vi "Read GMaps Attributes.vi"(0 "GMaps API in":refnum<class "GMaps API.lvclass">, 5 "error in (no error)":errorcluster) -> (14 "GMaps API out":refnum<class "GMaps API.lvclass">, 15 "GMaps Attributes":T1, 19 "error out":errorcluster)   [LabVIEW 2016, in "GMaps API.lvclass"]
doc: "Reads GMaps configured request."
uses:
  GMaps API.lvclass
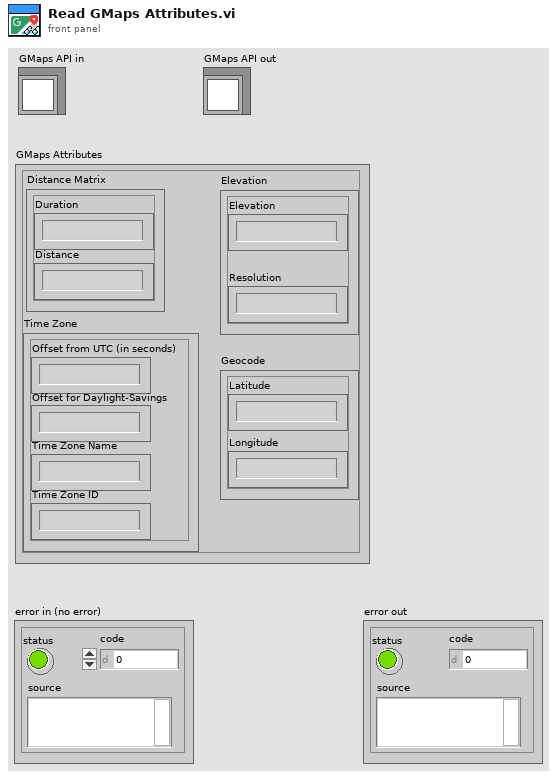
[diagram p1: front panel]
types:
  T1 = cluster{"Distance Matrix":cluster{"Duration":string, "Distance":string}, "Time Zone":cluster{"Offset from UTC (in seconds)":string, "Offset for Daylight-Savings":string, "Time Zone Name":string, "Time Zone ID":string}, "Elevation":cluster{"Elevation":string, "Resolution":string}, "Geocode":cluster{"Latitude":string, "Longitude":string}}
  T2 = cluster{"Offset for Daylight-Savings":string, "Offset from UTC (in seconds)":string, "Time Zone Name":string, "Time Zone ID":string}
  T3 = cluster{"Distance Matrix":cluster{"Duration":string, "Distance":string}, "Time Zone":cluster{"Offset for Daylight-Savings":string, "Offset from UTC (in seconds)":string, "Time Zone Name":string, "Time Zone ID":string}, "Elevation":cluster{"Elevation":string, "Resolution":string}, "Geocode":cluster{"Latitude":string, "Longitude":string}}
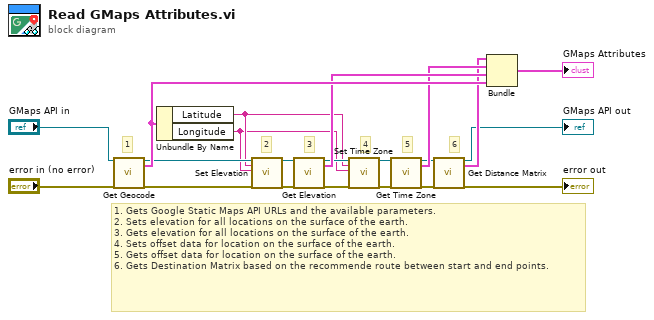
[diagram p0: block diagram]
diagram:
  # "1. Gets Google Static Maps API URLs and the available parameters.\n2. Sets elevation for all locations on the surface of the earth. \n3. Gets elevation for all locations on the surface of the earth. \n4. Sets offset data for location on the surface of the earth.\n5. Gets offset data for location on the surface of the earth.\n6. Gets Destination Matrix based on the recommende route between start and end points."
  # "6"
  # "5"
  # "4"
  # "3"
  # "2"
  # "1"
  n1 = call "Get Geocode.vi"("GMaps API in"="GMaps API in", "error in (no error)"="error in (no error)") -> ("GMaps API out"=w9:refnum<class "GMaps API.lvclass">, "Geocode"=w20:cluster{"Latitude":string, "Longitude":string}, "error out"=w13:errorcluster)  [unwired: 15 in]
  n2 = Unbundle By Name(w20) -> ("Latitude"=w2:string, "Longitude"=w1:string)
  n3 = call "Set Elevation.vi"("GMaps API in"=w9, "Latitude"=w2, "Longitude"=w1, "error in (no error)"=w13) -> ("GMaps API out"=w10:refnum<class "GMaps API.lvclass">, "error out"=w11:errorcluster)  [unwired: 14 in]
  n4 = call "Get Elevation.vi"("GMaps API in"=w10, "error in (no error)"=w11) -> ("GMaps API out"=w14:refnum<class "GMaps API.lvclass">, "Elevation"=w19:cluster{"Elevation":string, "Resolution":string}, "error out"=w12:errorcluster)  [unwired: 15 in]
  n5 = call "Set Time Zone.vi"("GMaps API in"=w14, "Latitude"=w2, "Longitude"=w1, "error in (no error)"=w12) -> ("GMaps API out"=w7:refnum<class "GMaps API.lvclass">, "error out"=w8:errorcluster)  [unwired: 14 in]
  n6 = call "Get Time Zone.vi"("GMaps API in"=w7, "error in (no error)"=w8) -> ("GMaps API out"=w15:refnum<class "GMaps API.lvclass">, "Time Zone"=w18:T2, "error out"=w16:errorcluster)  [unwired: 15 in]
  n7 = call "Get Distance Matrix.vi"("GMaps API in"=w15, "error in (no error)"=w16) -> ("GMaps API out"=→"GMaps API out":refnum<class "GMaps API.lvclass">, "Distance Matrix"=w17:cluster{"Duration":string, "Distance":string}, "error out"=→"error out":errorcluster)  [unwired: 15 in]
  n8 = Bundle("Distance Matrix"=w17, "Time Zone"=w18, "Elevation"=w19, "Geocode"=w20) -> (→"GMaps Attributes":T3)  [unwired: 1 in]
